vi "convert to 16 bit and save.vi"(9 "input array":dbl[][](array[numeric]), 11 "refnum in":refnum<file>) -> (3 "refnum out":refnum<file>)   [LabVIEW 2018]
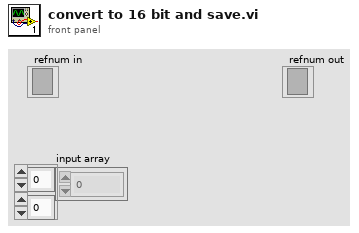
[diagram p1: front panel]
types:
  T1 = enum16{"big-endian, network order", "native, host order", "little-endian"}
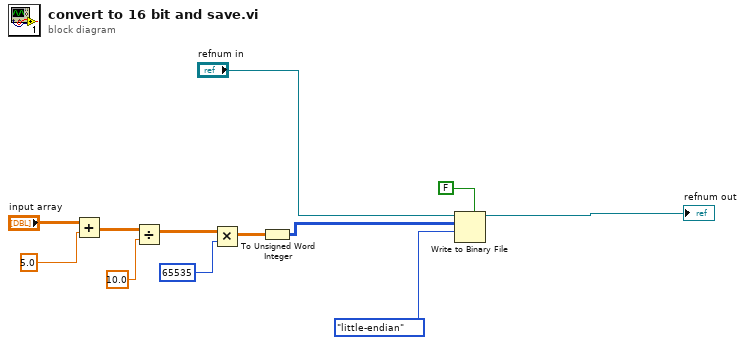
[diagram p0: block diagram]
diagram:
  n1 = Add(x="input array", y=5.0) -> (x+y=w6:dbl[][])
  n2 = Divide(x=w6, y=10.0) -> (x/y=w4:dbl[][])
  n3 = Multiply(x=w4, y=u16 65535) -> (x*y=w2:dbl[][])
  n4 = To Unsigned Word Integer(number=w2) -> (unsigned 16bit integer=w1:u16[][])
  n5 = Write to Binary File(file (use dialog)="refnum in", data=w1, 5:FALSE ("prepend array or string size? (T)"), 9:T1."little-endian" ("byte order (0:big-endian, network order)")) -> (refnum out=→"refnum out":refnum<file>)  [unwired: 2 in, 2 out]
